vi "data insert.vi"(8 "error in (no error)":errorcluster, 11 "data in":T1={"时间"=timestamp(0 s since 1904-01-01), "参数"="", "数据类型"="N", "加标前水样测试时间"=timestamp(0 s since 1904-01-01), "加标前水样浓度值"=0.0, "加标后水样浓度值"=0.0, "加标母液浓度值"=0.0, "加标体积"=0.0, "加标水杯定容体积"=0.0, "加标回收率"=0.0}) -> (0 "error out":errorcluster)   [LabVIEW 2016, in "质控单元V4.lvlib"]
uses:
  <vilib>/addons/database/Auxilliary.llb/DB Tools Column Info.ctl
  <vilib>/addons/database/Auxilliary.llb/DB Tools DataTypes.ctl
  <vilib>/addons/database/NI_Database_API.lvlib
  <vilib>/Utility/VariantDataType/VariantType.lvlib
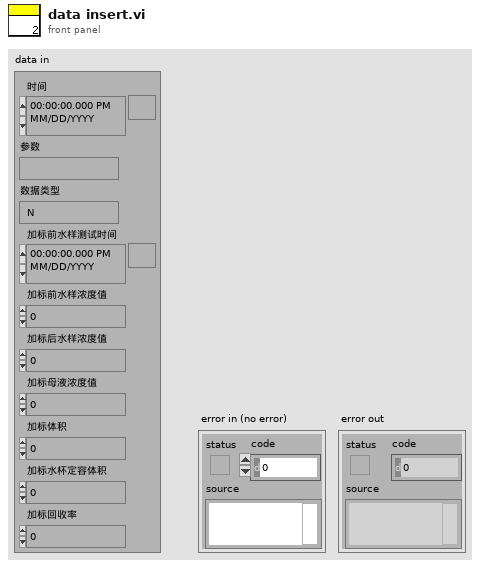
[diagram p1: front panel]
types:
  T1 = cluster{"时间":timestamp, "参数":string, "数据类型":string, "加标前水样测试时间":timestamp, "加标前水样浓度值":sgl, "加标后水样浓度值":sgl, "加标母液浓度值":sgl, "加标体积":sgl, "加标水杯定容体积":sgl, "加标回收率":sgl}
  T2 = typedef "NI_Database_API.lvlib/DB Tools Column Info.ctl" = cluster{"column name":string, "data type":T3, "size":i32, "allow null?":bool}
  T3 = typedef "NI_Database_API.lvlib/DB Tools DataTypes.ctl" = enum16{"String", "Long (I32)", "Single (SGL)", "Double (DBL)", "Date/Time", "Binary"}
  T4 = typedef "VariantType.lvlib/Type.ctl" = enum8{"Invalid Type", "Void", "I8", "I16", "I32", "I64", "U8", "U16", "U32", "U64", "Single Float", "Double Float", "Extended Float", "Single Complex", "Double Complex", "Extended Complex", "Enum U8", "Enum U16", "Enum U32", "Enum U64", "Single Float With Unit", "Double Float With Unit", "Extended Float With Unit", "Single Complex with Unit", "Double Complex with Unit", "Extended Complex with Unit", "Boolean", "String", "Path", "Picture", "Tag", "Array", "Cluster", "Variant", "LV Variant", "Waveform", "Timestamp", "Digital Waveform", "Digital Data", "ExpressData", "Refnum", "External Data", "VI", "Poly VI", "LabVIEW Class Instance", "Fixed Point"}
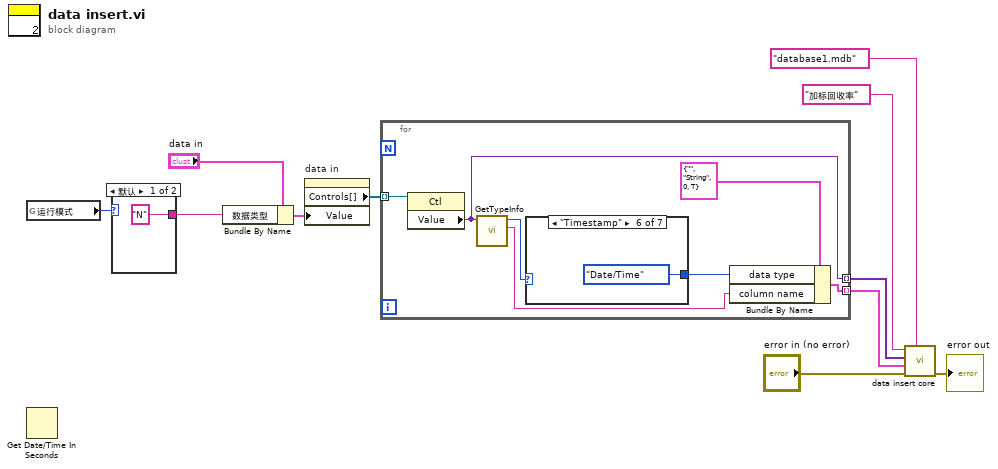
[diagram p0: block diagram]
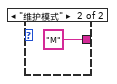
[diagram p2: hidden frame]
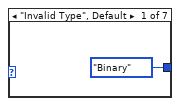
[diagram p3: hidden frame]
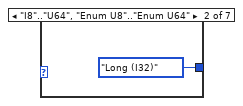
[diagram p4: hidden frame]
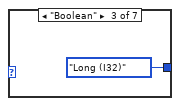
[diagram p5: hidden frame]
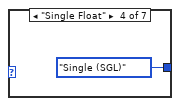
[diagram p6: hidden frame]
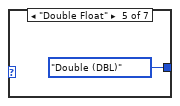
[diagram p7: hidden frame]
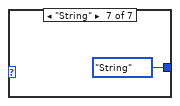
[diagram p8: hidden frame]
diagram:
  n1 = global read "系统交互.vi" "运行模式"() -> (w4:enum16{"维护模式", "常规模式", "应急模式", "质控模式"})
  n2 = Get Date/Time In Seconds() -> ()  [unwired: 1 out]
  n3 = case shown="默认" w4 {
    tunnel: ["N" "M"] -> w3
    frame Default {
    }
    frame "维护模式" {
    }
  }
  n4 = Bundle By Name(cluster="data in", "数据类型"=w3) -> (w5:T1)
  n5 = property on="data in" class="Clust (严格)"("Value"=w5) -> ("Controls[]"=w11:refnum<vi>[])  [unwired: 2 in, 2 out]
  n6 = for {
    tunnel: w11 -> [w20] mode=indexing
    tunnel: [w14] -> w2 mode=indexing
    tunnel: [w15] -> w8 mode=indexing
    n7 = property class="Ctl"(reference=w20) -> ("Value"=w14:variant)  [unwired: 1 in, 2 out]
    n8 = call <vilib>:"GetTypeInfo.vi"("Variant"=w14) -> ("Name"=w18:string, "Type Enum"=w17:T4)  [unwired: 6 in, 3 out]
    n9 = case shown="\"Timestamp\"" w17 {
      tunnel: [DB_Tools_DataTypes."Binary" ("data type") DB_Tools_DataTypes."Long (I32)" ("data type") DB_Tools_DataTypes."Long (I32)" ("data type") DB_Tools_DataTypes."Single (SGL)" ("data type") DB_Tools_DataTypes."Double (DBL)" ("data type") DB_Tools_DataTypes."Date/Time" ("data type") DB_Tools_DataTypes."String" ("data type")] -> w16
      frame "Invalid Type", Default {
      }
      frame "I8".."U64", "Enum U8".."Enum U64" {
      }
      frame "Boolean" {
      }
      frame "Single Float" {
      }
      frame "Double Float" {
      }
      frame "Timestamp" {
      }
      frame "String" {
      }
    }
    n10 = Bundle By Name(cluster=T2 {"column name"="", "data type"=enum."String", "size"=0, "allow null?"=TRUE} ("column information"), "data type"=w16, "column name"=w18) -> (w15:T2)
  }
  n11 = call "data insert core.vi"("database"="database1.mdb", "error in (no error)"="error in (no error)", "column information"=w8, "data"=w2, "table"="加标回收率") -> ("error out"=→"error out":errorcluster)  [unwired: 6 in]
